vi "Wiimote Get Core Buttons and Acceleration.vi"(8 "error in":errorcluster, 11 "hWiimoteHandle in":u32 format="%08x") -> (0 "error out":errorcluster, 1 "Wiimote Acceleration out":T1, 2 "Wiimote Buttons out":T2, 3 "hWiimoteHandle out":u32 format="%08x")   [LabVIEW 2011, in "Wiimote.lvlib"]
uses:
  Wiimote.lvlib
  Wiimote Buttons.ctl
  Wiimote Acceleration.ctl
  Wiimote Reporting Mode.ctl
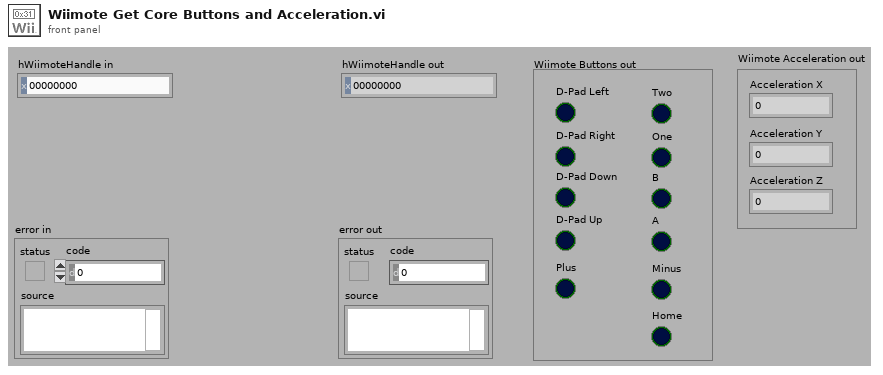
[diagram p1: front panel]
types:
  T1 = typedef "Wiimote.lvlib/Wiimote Acceleration.ctl" = cluster{"Acceleration X":dbl, "Acceleration Y":dbl, "Acceleration Z":dbl}
  T2 = typedef "Wiimote.lvlib/Wiimote Buttons.ctl" = cluster{"D-Pad Left":bool, "D-Pad Right":bool, "D-Pad Down":bool, "D-Pad Up":bool, "Plus":bool, "Two":bool, "One":bool, "B":bool, "A":bool, "Minus":bool, "Home":bool}
  T3 = typedef "Wiimote.lvlib/Wiimote Reporting Mode.ctl" = u8
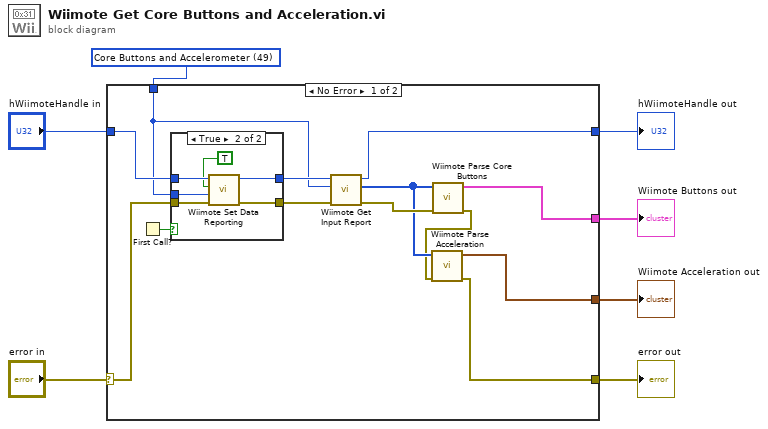
[diagram p0: block diagram]
diagram:
  w1 = T3 49 items=["Core Buttons"=48, "Core Buttons and Accelerometer"=49, "Core Buttons with 8 Extension bytes"=50, "Core Buttons and Accelerometer with 12 IR bytes"=51, "Core Buttons with 19 Extension bytes"=52, "Core Buttons and Accelerometer with 16 Extension Bytes"=53, "Core Buttons with 10 IR bytes and 9 Extension Bytes"=54, "Core Buttons and Accelerometer with 10 IR bytes and 6 Extension Bytes"=55] ("Reporting Mode")
  n1 = case shown="No Error" "error in" {
    selector: "error in" -> [w10 w30]
    tunnel: [w14 w30] -> w6
    tunnel: "hWiimoteHandle in" -> [w11 w29]
    tunnel: [w19 w29] -> w4
    tunnel: [w18 _] -> w3
    tunnel: [w16 _] -> w2
    tunnel: w1 -> [w8 _]
    frame No Error {
      n2 = First Call?() -> (First Call?: T/F=w9:bool)
      n3 = case shown="True" w9 {
        tunnel: [w22 w26] -> w13
        tunnel: [w21 w25] -> w12
        tunnel: w11 -> [w22 w28]
        tunnel: w10 -> [w21 w27]
        tunnel: w8 -> [_ w23]
        frame False {
        }
        frame True {
          n4 = call "Wiimote Set Data Reporting.vi"("error in"=w27, "Reporting Mode"=w23, "Continuous"=TRUE, "hWiimoteHandle in"=w28) -> ("error out"=w25:errorcluster, "hWiimoteHandle out"=w26:u32)  [unwired: 6 in]
        }
      }
      n5 = call "Wiimote Get Input Report.vi"("error in"=w12, "bInputReport"=w8, "hWiimoteHandle in"=w13) -> ("error out"=w20:errorcluster, "pReportBuffer out"=w17:u8[], "hWiimoteHandle out"=w19:u32)  [unwired: 6 in]
      n6 = call "Wiimote Parse Core Buttons.vi"("error in"=w20, "pReportBuffer in"=w17) -> ("error out"=w15:errorcluster, "Wiimote Buttons out"=w18:T2)  [unwired: 8 in]
      n7 = call "Wiimote Parse Acceleration.vi"("error in"=w15, "pReportBuffer in"=w17) -> ("error out"=w14:errorcluster, "Wiimote Acceleration Raw out"=w16:T1)  [unwired: 8 in]
    }
    frame Error {
    }
  }
  "error out" <- w6
  "hWiimoteHandle out" <- w4
  "Wiimote Buttons out" <- w3
  "Wiimote Acceleration out" <- w2
